vi "Launch Freezer.vi"(7 "Freezer":T1=enum."Syringe", 8 "error in (no error)":errorcluster, 11 "cRIO-CO2 in":refnum<class "cRIO-CO2.lvclass">) -> (0 "error out":errorcluster, 3 "cRIO-CO2 out":refnum<class "cRIO-CO2.lvclass">)   [LabVIEW 2015, in "cRIO-Carbondioxide.lvlib" / "cRIO-CO2.lvlib" / "cRIO-CO2.lvclass"]
uses:
  cRIO-CO2.lvclass
  Freezers Enumerator.ctl
  <vilib>/ActorFramework/Actor/Actor.lvclass
  cRIO-CO2.lvclass/cRIO-CO2.ctl
  cRIO-CO2 Messages/Log Message Msg/Log Message Msg.lvclass/Log Message Msg.ctl
  <vilib>/ActorFramework/Message Enqueuer/Message Enqueuer.lvclass/Message Enqueuer.ctl
  Blowers Heaters Enumerator.ctl
  <vilib>/ActorFramework/Message Enqueuer/Enqueue.vi
  <vilib>/ActorFramework/Message Priority Queue/Priority Enqueue.vi
  <vilib>/ActorFramework/Message Enqueuer/Message Enqueuer.lvclass
  cRIO-CO2 Messages/Log Message Msg/Log Message Msg.lvclass
  Freezer/Freezer.lvclass
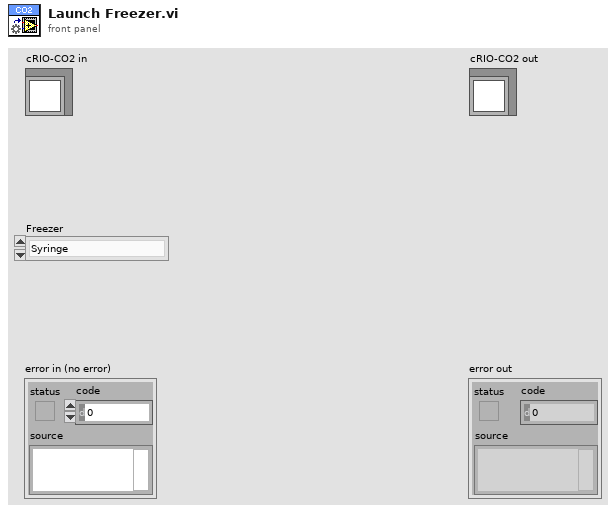
[diagram p1: front panel]
types:
  T1 = typedef "cRIO-Carbondioxide.lvlib/cRIO-CO2.lvlib/cRIO-CO2.lvclass/Freezers Enumerator.ctl" = enum16{"Undefined", "Syringe", "Cold Tank 1", "Cold Tank 2", "Cold Tank 3", "Cold Tank 4"}
  T2 = cluster{"Switch SHV":refnum<k21>, "Thermocouple SHV":refnum<k21>, "LN Valve SHV":refnum<k21>}
  T3 = typedef "cRIO-Carbondioxide.lvlib/cRIO-CO2.lvlib/cRIO-CO2.lvclass/Blowers Heaters Enumerator.ctl" = enum16{"Tank Blower 1", "Tank Blower 2", "Tank Blower 3", "Tank Blower 4", "Syringe Blower", "Syringe Heater", "Piston Heater", "Undefined"}
  T4 = typedef "Dedicated Enqueuers.ctl" = cluster{"Freezers":cluster{"Syringe":refnum<class "Message Enqueuer.lvclass">, "Tank 1":refnum<class "Message Enqueuer.lvclass">, "Tank 2":refnum<class "Message Enqueuer.lvclass">, "Tank 3":refnum<class "Message Enqueuer.lvclass">, "Tank 4":refnum<class "Message Enqueuer.lvclass">}, "Heaters":cluster{"Syringe":refnum<class "Message Enqueuer.lvclass">, "Piston":refnum<class "Message Enqueuer.lvclass">}, "Blowers":cluster{"Tank 1":refnum<class "Message Enqueuer.lvclass">, "Tank 2":refnum<class "Message Enqueuer.lvclass">, "Tank 3":refnum<class "Message Enqueuer.lvclass">, "Tank 4":refnum<class "Message Enqueuer.lvclass">, "Syringe":refnum<class "Message Enqueuer.lvclass">}, "Sample Line":refnum<class "Message Enqueuer.lvclass">, "Storage Line":refnum<class "Message Enqueuer.lvclass">, "Transfer Line":refnum<class "Message Enqueuer.lvclass">, "Syringe Stepper":refnum<class "Message Enqueuer.lvclass">, "Syringe Line":refnum<class "Message Enqueuer.lvclass">, "Capillary Line":refnum<class "Message Enqueuer.lvclass">, "Preparation Line":refnum<class "Message Enqueuer.lvclass">, "Turbo":refnum<class "Message Enqueuer.lvclass">, "Vacuum":refnum<class "Message Enqueuer.lvclass">, "He Line":refnum<class "Message Enqueuer.lvclass">, "Cylinder":refnum<class "Message Enqueuer.lvclass">}
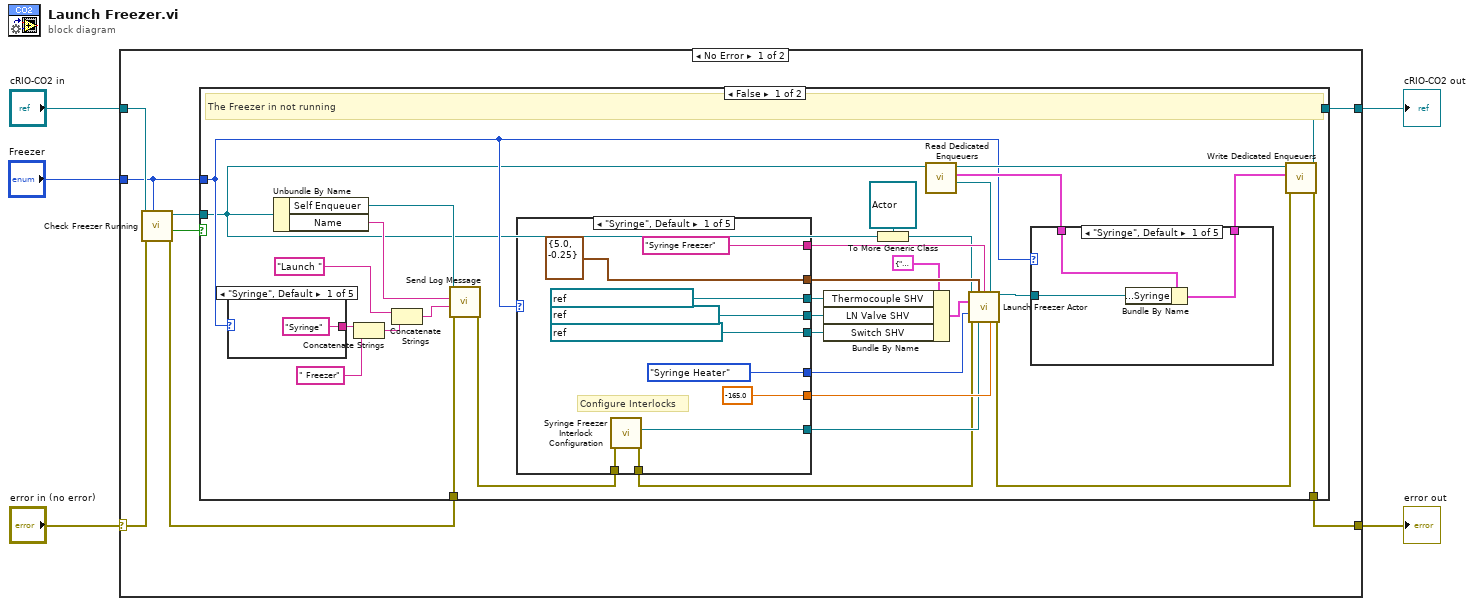
[diagram p0: block diagram]
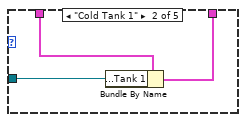
[diagram p2: hidden frame]
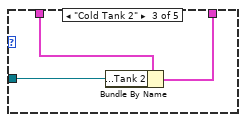
[diagram p3: hidden frame]
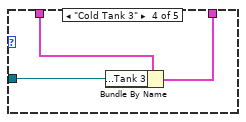
[diagram p4: hidden frame]
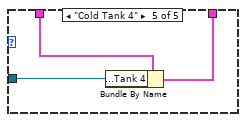
[diagram p5: hidden frame]
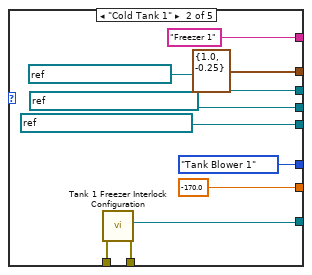
[diagram p6: hidden frame]
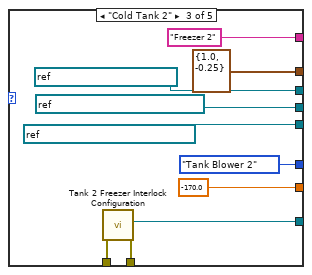
[diagram p7: hidden frame]
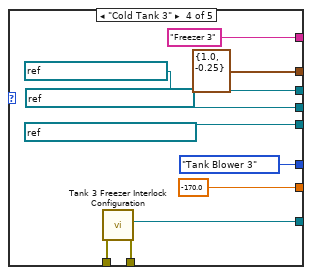
[diagram p8: hidden frame]
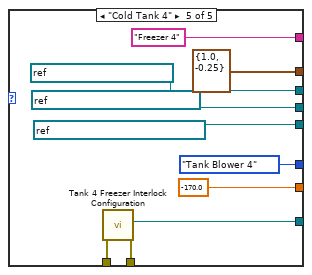
[diagram p9: hidden frame]
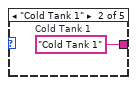
[diagram p10: hidden frame]
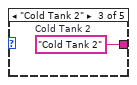
[diagram p11: hidden frame]
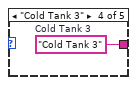
[diagram p12: hidden frame]
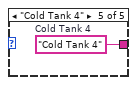
[diagram p13: hidden frame]
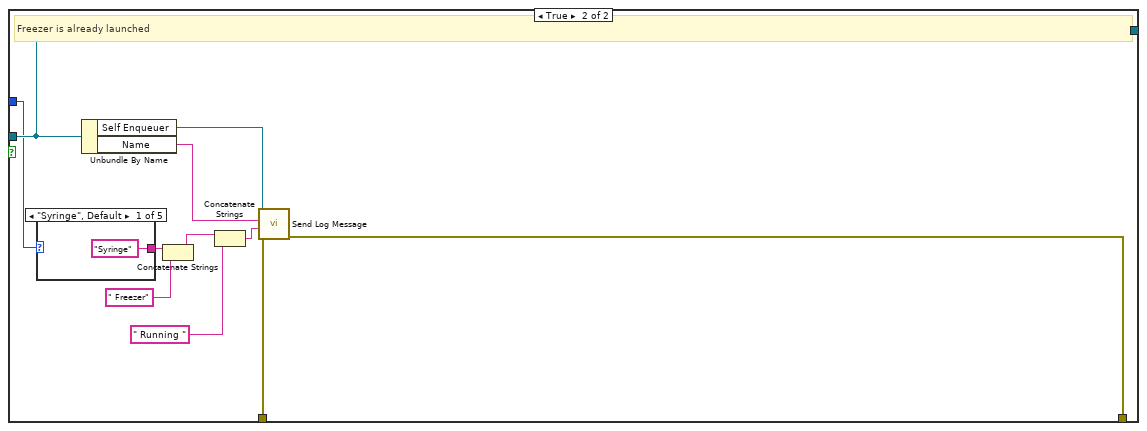
[diagram p14: hidden frame]
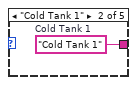
[diagram p15: hidden frame]
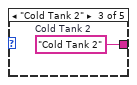
[diagram p16: hidden frame]
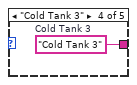
[diagram p17: hidden frame]
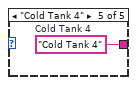
[diagram p18: hidden frame]
diagram:
  n1 = case shown="No Error" "error in (no error)" {
    selector: "error in (no error)" -> [w11 w133]
    tunnel: [w6 w133] -> w4
    tunnel: [w8 w132] -> w2
    tunnel: "cRIO-CO2 in" -> [w13 w132]
    tunnel: "Freezer" -> [w12 _]
    frame No Error {
      n2 = call "Check Freezer Running.vi"("Freezer"=w12, "error in (no error)"=w11, "cRIO-CO2 in"=w13) -> ("error out"=w10:errorcluster, "Running?"=w9:bool, "cRIO-CO2 out"=w7:refnum<class "cRIO-CO2.lvclass">)  [unwired: 6 in]
      n3 = case shown="False" w9 {
        tunnel: w7 -> [w20 w118]
        tunnel: w12 -> [w22 w117]
        tunnel: w10 -> [w29 w122]
        tunnel: [w25 w118] -> w8
        tunnel: [w14 w116] -> w6
        frame False {
          # "The Freezer in not running"
          n4 = case shown="\"Syringe\", Default" w22 {
            tunnel: ["Syringe" w112 w113 w114 w115] -> w44
            frame "Syringe", Default {
            }
            frame "Cold Tank 1" {
              w112 = "Cold Tank 1"  # Cold Tank 1
            }
            frame "Cold Tank 2" {
              w113 = "Cold Tank 2"  # Cold Tank 2
            }
            frame "Cold Tank 3" {
              w114 = "Cold Tank 3"  # Cold Tank 3
            }
            frame "Cold Tank 4" {
              w115 = "Cold Tank 4"  # Cold Tank 4
            }
          }
          n5 = Unbundle By Name(w20) -> ("Self Enqueuer"=w39:refnum<class "Message Enqueuer.lvclass">, "Name"=w45:string)
          n6 = Concatenate Strings(w44, " Freezer" ("string")) -> (w42:string)
          n7 = Concatenate Strings("Launch " ("String"), w42) -> (w40:string)
          n8 = call "Send Log Message.vi"("error in (no error)"=w29, "String"=w40, "Source Name"=w45, "Message Enqueuer"=w39) -> ("error out"=w28:errorcluster)  [unwired: 6 in, 1 out]
          n9 = case shown="\"Syringe\", Default" w22 {
            tunnel: [cluster{"Upper":dbl, "Lower":dbl} {"Upper"=5.0, "Lower"=-0.25} ("Thresholds") cluster{"Upper":dbl, "Lower":dbl} {"Upper"=1.0, "Lower"=-0.25} ("Thresholds") cluster{"Upper":dbl, "Lower":dbl} {"Upper"=1.0, "Lower"=-0.25} ("Thresholds") cluster{"Upper":dbl, "Lower":dbl} {"Upper"=1.0, "Lower"=-0.25} ("Thresholds") cluster{"Upper":dbl, "Lower":dbl} {"Upper"=1.0, "Lower"=-0.25} ("Thresholds")] -> w38
            tunnel: [refnum<k21> "ni.var.psp://10.2.0.20/AMS Gas SHV/Gauges/Syringe TC" ("Thermocouple SHV") refnum<k21> "ni.var.psp://10.2.0.20/AMS Gas SHV/Gauges/Cold Tank TC 1" ("Thermocouple SHV") refnum<k21> "ni.var.psp://10.2.0.20/AMS Gas SHV/Gauges/Cold Tank TC 2" ("Thermocouple SHV") refnum<k21> "ni.var.psp://10.2.0.20/AMS Gas SHV/Gauges/Cold Tank TC 3" ("Thermocouple SHV") refnum<k21> "ni.var.psp://10.2.0.20/AMS Gas SHV/Gauges/Cold Tank TC 4" ("Thermocouple SHV")] -> w34
            tunnel: [refnum<k21> "ni.var.psp://10.2.0.20/AMS Gas SHV/Valves/LN Feed Valves/Cold Tank Syringe" ("LN Valve SHV") refnum<k21> "ni.var.psp://10.2.0.20/AMS Gas SHV/Valves/LN Feed Valves/Cold Tank Storage 1" ("LN Valve SHV") refnum<k21> "ni.var.psp://10.2.0.20/AMS Gas SHV/Valves/LN Feed Valves/Cold Tank Storage 2" ("LN Valve SHV") refnum<k21> "ni.var.psp://10.2.0.20/AMS Gas SHV/Valves/LN Feed Valves/Cold Tank Storage 3" ("LN Valve SHV") refnum<k21> "ni.var.psp://10.2.0.20/AMS Gas SHV/Valves/LN Feed Valves/Cold Tank Storage 4" ("LN Valve SHV")] -> w33
            tunnel: [-165.0 ("Low Temp (-170)") -170.0 ("Low Temp (-170)") -170.0 ("Low Temp (-170)") -170.0 ("Low Temp (-170)") -170.0 ("Low Temp (-170)")] -> w37
            tunnel: [refnum<k21> "ni.var.psp://10.2.0.20/AMS Gas SHV/Freezers/Freezer Syringe" ("Switch SHV") refnum<k21> "ni.var.psp://10.2.0.20/AMS Gas SHV/Freezers/Freezer Tank 1" ("Switch SHV") refnum<k21> "ni.var.psp://10.2.0.20/AMS Gas SHV/Freezers/Freezer Tank 2" ("Switch SHV") refnum<k21> "ni.var.psp://10.2.0.20/AMS Gas SHV/Freezers/Freezer Tank 3" ("Switch SHV") refnum<k21> "ni.var.psp://10.2.0.20/AMS Gas SHV/Freezers/Freezer Tank 4" ("Switch SHV")] -> w32
            tunnel: ["Syringe Freezer" ("Name") "Freezer 1" ("Name") "Freezer 2" ("Name") "Freezer 3" ("Name") "Freezer 4" ("Name")] -> w36
            tunnel: w28 -> [w65 w74 w84 w94 w104]
            tunnel: [w64 w73 w83 w93 w103] -> w16
            tunnel: [w63 w72 w82 w92 w102] -> w30
            tunnel: [Blowers_Heaters_Enumerator."Syringe Heater" ("Heater") Blowers_Heaters_Enumerator."Tank Blower 1" ("Heater") Blowers_Heaters_Enumerator."Tank Blower 2" ("Heater") Blowers_Heaters_Enumerator."Tank Blower 3" ("Heater") Blowers_Heaters_Enumerator."Tank Blower 4" ("Heater")] -> w19
            frame "Syringe", Default {
              # "Configure Interlocks"
              n10 = call "Syringe Freezer Interlock Configuration.vi"("error in (no error)"=w65) -> ("error out"=w64:errorcluster, "Interlock Chain"=w63:refnum<class "Interlock Chain.lvclass">)  [unwired: 8 in, 1 out]
            }
            frame "Cold Tank 1" {
              n11 = call "Tank 1 Freezer Interlock Configuration.vi"("error in (no error)"=w74) -> ("error out"=w73:errorcluster, "Interlock Chain"=w72:refnum<class "Interlock Chain.lvclass">)  [unwired: 8 in, 1 out]
            }
            frame "Cold Tank 2" {
              n12 = call "Tank 2 Freezer Interlock Configuration.vi"("error in (no error)"=w84) -> ("error out"=w83:errorcluster, "Interlock Chain"=w82:refnum<class "Interlock Chain.lvclass">)  [unwired: 8 in, 1 out]
            }
            frame "Cold Tank 3" {
              n13 = call "Tank 3 Freezer Interlock Configuration.vi"("error in (no error)"=w94) -> ("error out"=w93:errorcluster, "Interlock Chain"=w92:refnum<class "Interlock Chain.lvclass">)  [unwired: 8 in, 1 out]
            }
            frame "Cold Tank 4" {
              n14 = call "Tank 4 Freezer Interlock Configuration.vi"("error in (no error)"=w104) -> ("error out"=w103:errorcluster, "Interlock Chain"=w102:refnum<class "Interlock Chain.lvclass">)  [unwired: 8 in, 1 out]
            }
          }
          n15 = Bundle By Name(cluster=T2 {"Switch SHV"="", "Thermocouple SHV"="", "LN Valve SHV"=""} ("SHVs"), "Thermocouple SHV"=w34, "LN Valve SHV"=w33, "Switch SHV"=w32) -> (w31:T2)
          n16 = To More Generic Class(target class=refnum<class "Actor.lvclass"> refnum ("Caller Actor in"), reference=w20) -> (generic class reference=w18:refnum<class "Actor.lvclass">)
          n17 = call "Read Dedicated Enqueuers.vi"("cRIO-CO2 in"=w20) -> ("Qs.DedicatedEnQrs"=w17:refnum<queue>, "Dedicated Enqueuers"=w24:T4, "cRIO-CO2 out"=w26:refnum<class "cRIO-CO2.lvclass">)  [unwired: 7 in, 1 out]
          n18 = call "Launch Freezer Actor.vi"("Caller Actor in"=w18, "Thresholds"=w38, "Name"=w36, "DedicatedEnQrs"=w17, "SHVs"=w31, "Heater"=w19, "error in (no error)"=w16, "Interlock Chain"=w30, "Low Temp (-170)"=w37) -> ("Caller-To-Actor Enqueuer"=w27:refnum<class "Message Enqueuer.lvclass">, "error out"=w15:errorcluster)  [unwired: 5 in]
          n19 = case shown="\"Syringe\", Default" w22 {
            tunnel: w24 -> [w48 w51 w54 w57 w60]
            tunnel: w27 -> [w47 w50 w53 w56 w59]
            tunnel: [w46 w49 w52 w55 w58] -> w23
            frame "Syringe", Default {
              n20 = Bundle By Name(cluster=w48, "Freezers.Syringe"=w47) -> (w46:T4)
            }
            frame "Cold Tank 1" {
              n21 = Bundle By Name(cluster=w51, "Freezers.Tank 1"=w50) -> (w49:T4)
            }
            frame "Cold Tank 2" {
              n22 = Bundle By Name(cluster=w54, "Freezers.Tank 2"=w53) -> (w52:T4)
            }
            frame "Cold Tank 3" {
              n23 = Bundle By Name(cluster=w57, "Freezers.Tank 3"=w56) -> (w55:T4)
            }
            frame "Cold Tank 4" {
              n24 = Bundle By Name(cluster=w60, "Freezers.Tank 4"=w59) -> (w58:T4)
            }
          }
          n25 = call "Write Dedicated Enqueuers.vi"("error in (no error)"=w15, "Dedicated Enqueuers"=w23, "cRIO-CO2 in"=w26) -> ("error out"=w14:errorcluster, "cRIO-CO2 out"=w25:refnum<class "cRIO-CO2.lvclass">)  [unwired: 7 in]
        }
        frame True {
          # "Freezer is already launched"
          n26 = case shown="\"Syringe\", Default" w117 {
            tunnel: ["Syringe" w128 w129 w130 w131] -> w125
            frame "Syringe", Default {
            }
            frame "Cold Tank 1" {
              w128 = "Cold Tank 1"  # Cold Tank 1
            }
            frame "Cold Tank 2" {
              w129 = "Cold Tank 2"  # Cold Tank 2
            }
            frame "Cold Tank 3" {
              w130 = "Cold Tank 3"  # Cold Tank 3
            }
            frame "Cold Tank 4" {
              w131 = "Cold Tank 4"  # Cold Tank 4
            }
          }
          n27 = Unbundle By Name(w118) -> ("Self Enqueuer"=w123:refnum<class "Message Enqueuer.lvclass">, "Name"=w126:string)
          n28 = Concatenate Strings(w125, " Freezer" ("string")) -> (w121:string)
          n29 = Concatenate Strings(w121, " Running " ("String")) -> (w119:string)
          n30 = call "Send Log Message.vi"("error in (no error)"=w122, "String"=w119, "Source Name"=w126, "Message Enqueuer"=w123) -> ("error out"=w116:errorcluster)  [unwired: 6 in, 1 out]
        }
      }
    }
    frame Error {
    }
  }
  "error out" <- w4
  "cRIO-CO2 out" <- w2
